vi "TSCAN_Receive.vi"(7 "错误输入（无错误）":errorcluster, 8 "读取报文类型":u16(ring) items=["只读取接收报文", "发送报文&接收报文"], 9 "AAPPChannel":u32, 10 "路径输入":path) -> (0 "错误输出":errorcluster, 2 "ACANMsgBuffer":T1(array[cluster]), 3 "路径输出":path)   [LabVIEW 2019]
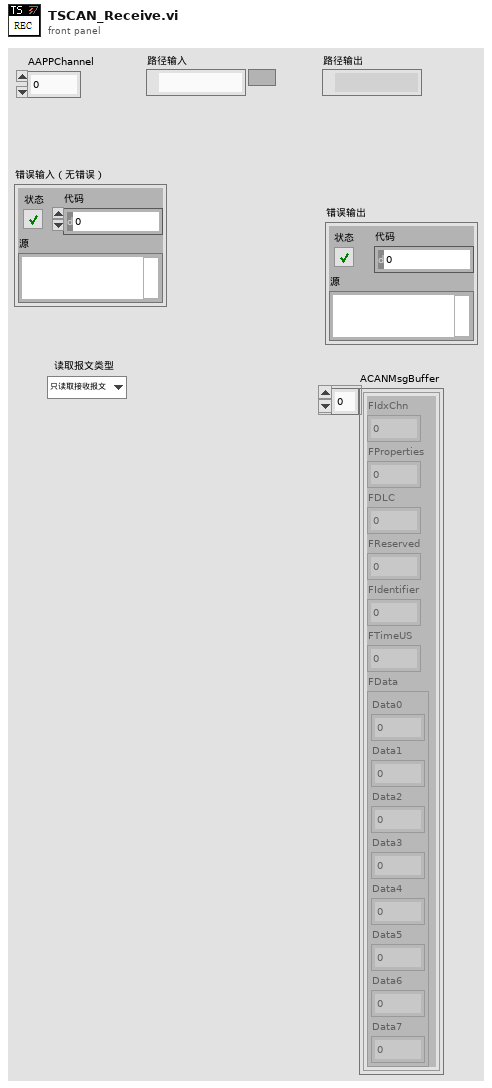
[diagram p1: front panel]
types:
  T1 = cluster{"FIdxChn":u8, "FProperties":u8, "FDLC":u8, "FReserved":u8, "FIdentifier":i32, "FTimeUS":u64, "FData":cluster{"Data0":u8, "Data1":u8, "Data2":u8, "Data3":u8, "Data4":u8, "Data5":u8, "Data6":u8, "Data7":u8}}[]
  T2 = cluster{"FIdxChn":u8, "FProperties":u8, "FDLC":u8, "FReserved":u8, "FIdentifier":i32, "FTimeUS":u64, "FData":cluster{"Data0":u8, "Data1":u8, "Data2":u8, "Data3":u8, "Data4":u8, "Data5":u8, "Data6":u8, "Data7":u8}}
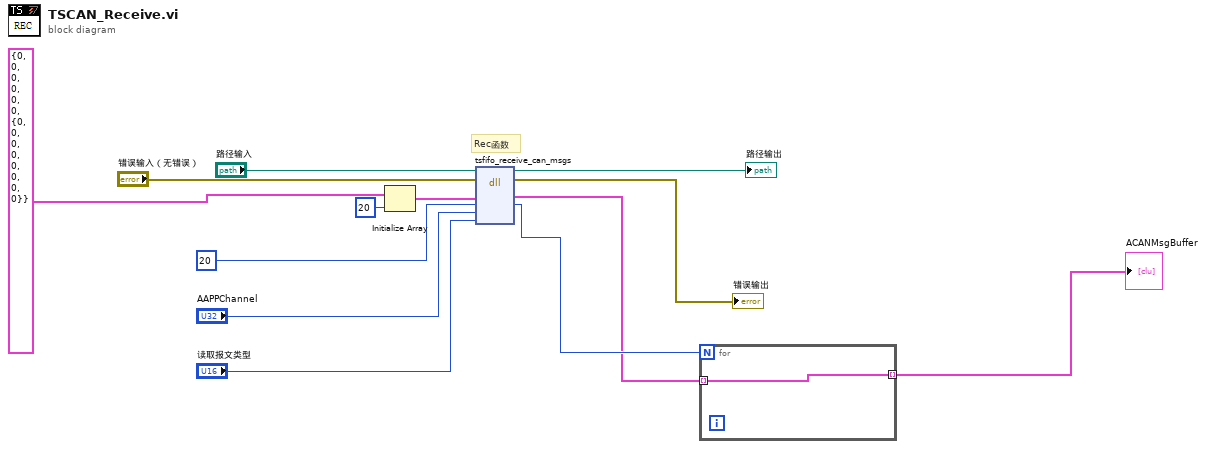
[diagram p0: block diagram]
diagram:
  # "Rec函数"
  n1 = Initialize Array(T2 {"FIdxChn"=0, "FProperties"=0, "FDLC"=0, "FReserved"=0, "FIdentifier"=0, "FTimeUS"=0, "FData"={"Data0"=0, "Data1"=0, "Data2"=0, "Data3"=0, "Data4"=0, "Data5"=0, "Data6"=0, "Data7"=0}} ("簇"), 20 ("维数大小")) -> (w13:T1)
  n2 = dll-call lib="PTH2Habs CUsers\nAdministratorDesktopTS_Can通讯PathTSMaster.dll" fn="tsfifo_receive_can_msgs"(path in="路径输入", error in="错误输入（无错误）", "ACANMsgBuffer"=w13, "ACANMsgBufferSize"=20, "AChn"="AAPPChannel", "ATxRx"="读取报文类型") -> (path out=→"路径输出":path, error out=→"错误输出":errorcluster, "ACANMsgBuffer"=w2:T1, "ACANMsgBufferSize"=w3:i32)  [unwired: 4 in]
  n3 = for {
    N: w3 -> [_]
    tunnel: w2 -> [w14] mode=indexing
    tunnel: [w14] -> w1 mode=indexing
  }
  "ACANMsgBuffer" <- w1
